vi "ProiectIV.vi"() -> ()   [LabVIEW 2020]
uses:
  65261286-63d7-44c7-95d4-ed37a7534505.vi
  <vilib>/MakerHub/LINX/Public/Peripherals/Digital/Digital Write 1 Chan.vi
  <vilib>/MakerHub/LINX/Public/Peripherals/PWM/PWM Set Duty Cycle 1 Chan.vi
  <vilib>/MakerHub/LINX/Public/Peripherals/Digital/Digital Write N Chans.vi
  <vilib>/MakerHub/LINX/Private/Local IO/LinxDigitalWrite.vi
  <vilib>/MakerHub/LINX/Public/Utilities/Check Channel.vi
  <vilib>/MakerHub/LINX/Public/Utilities/Open Serial.vi
  <vilib>/MakerHub/LINX/Private/Utilties/Generate Error.vi
  <vilib>/MakerHub/LINX/Public/Peripherals/PWM/PWM Set Duty Cycle N Chans.vi
  <vilib>/Comparison/Equal/Equal Functor/Equal Functor.lvclass
  <vilib>/MakerHub/LINX/LMH-LINX.lvlib
panel:
  out "UID Password":string
  out "UID vizibil":string
  out "?":string="Va rugam apropiati cardul"
  out "Nu se permite accesul":bool
  out "Se permite accesul":bool
  in  "Buton de oprire a programului":bool
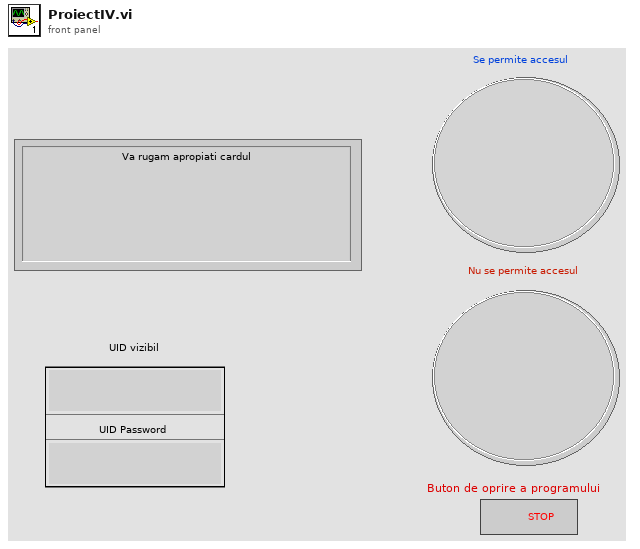
[diagram p1: front panel]
types:
  T1 = typedef "LMH-LINX.lvlib/LINX Ref.ctl" = cluster{"IO":T2, "Interface":T3, "LINX Device Config":T4}
  T2 = typedef "LMH-LINX.lvlib/Platform.ctl" = enum16{"Remote", "Local"}
  T3 = typedef "LMH-LINX.lvlib/Interface.ctl" = enum16{"Serial", "TCP"}
  T4 = typedef "LMH-LINX.lvlib/Device.lvlib/LINX Device Config.ctl" = cluster{"Interface":T3, "COM Port":refnum<visa-resource-name>, "TCP Configuration":T5, "Device Family":u8, "Device ID":u8, "Device Name":string, "TCP Ref":refnum<k5>, "Channels":T6}
  T5 = typedef "LMH-LINX.lvlib/Device.lvlib/TCP Config.ctl" = cluster{"IP Address":string, "Port":u16}
  T6 = typedef "LMH-LINX.lvlib/Channels.ctl" = cluster{"DI":u8[], "DO":u8[], "AI":u8[], "AO":u8[], "PWM":u8[], "QE":u8[], "UART":u8[], "I2C 2":u8[], "SPI":u8[], "CAN":u8[], "Servo":u8[], "AI Ref (V)":dbl, "AI Resolution (Bits)":u8, "AO Ref (V)":dbl, "AO Resolution (Bits)":u8}
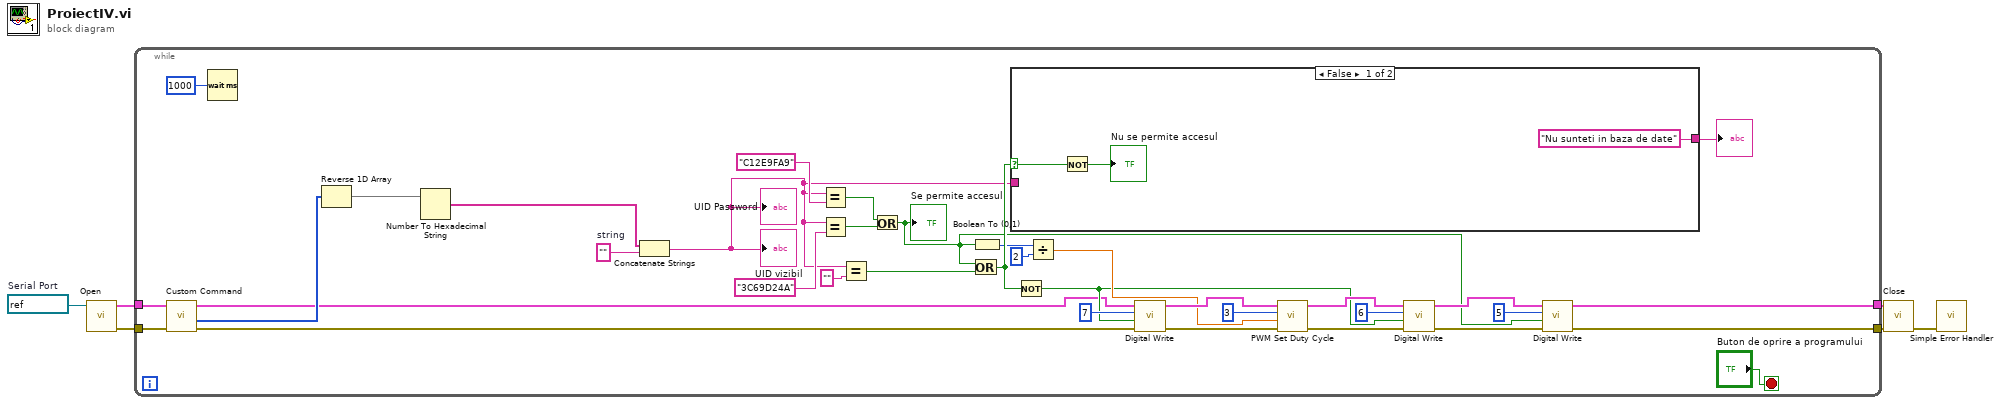
[diagram p0: block diagram]
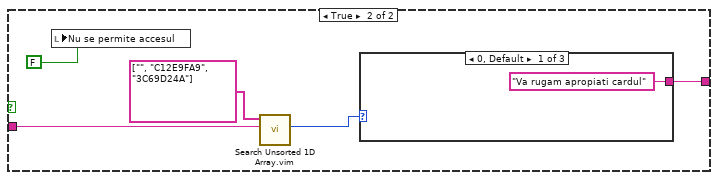
[diagram p2: hidden frame]
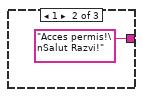
[diagram p3: hidden frame]
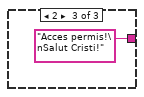
[diagram p4: hidden frame]
diagram:
  w3 = refnum<visa-resource-name> "COM3"  # Serial Port
  n1 = call-poly <vilib>:"Open.vi"("Serial Port"=w3) -> ("Error Out"=w5:errorcluster, "LINX Resource"=w6:T1)  [unwired: 8 in, 1 out]
  n2 = while {
    tunnel: w6 -> [w42]
    tunnel: w5 -> [w41]
    tunnel: [w12] -> w2
    tunnel: [w11] -> w1
    stop <- "Buton de oprire a programului" stop-if-true
    w37 = ""  # string
    n3 = call <vilib>:"Custom Command.vi"("Error In"=w41, "LINX Resource"=w42) -> ("Error Out"=w28:errorcluster, "Response"=w40:u8[], "LINX Resource"=w8:T1)  [unwired: 6 in, 1 out]
    n4 = Wait (ms)(milliseconds to wait=u32 1000) -> ()  [unwired: 1 out]
    n5 = Reverse 1D Array(array=w40) -> (reversed array=w32:u8[])
    n6 = Number To Hexadecimal String(2:w32) -> (0:w38:string[])  [unwired: 1 in]
    n7 = Concatenate Strings "Concatenate Strings"(w38, w37) -> (w7:string)
    "UID vizibil" <- w7
    "UID Password" <- w7
    n8 = Equal?(x=w7, y="C12E9FA9" ("false string")) -> (x = y?=w31:bool)
    n9 = Equal?(x=w7, y="3C69D24A") -> (x = y?=w33:bool)
    n10 = Equal?(x=w7, y="") -> (x = y?=w29:bool)
    n11 = Or(x=w31, y=w33) -> (x .or. y?=w9:bool)
    "Se permite accesul" <- w9
    n12 = Or(x=w9, y=w29) -> (x .or. y?=w26:bool)
    n13 = Boolean To (0,1)(Boolean=w9) -> (0, 1=w21:i16)
    n14 = case shown="False" w26 {
      selector: w26 -> [w43 _]
      tunnel: ["Nu sunteti in baza de date" w48] -> w25
      tunnel: w7 -> [_ w47]
      frame False {
        n15 = Not(x=w43) -> (.not. x?=→"Nu se permite accesul":bool)
      }
      frame True {
        n16 = local write "Nu se permite accesul"(FALSE ("Boolean 3")) -> ()
        n17 = call "Search Unsorted 1D Array.vim"("element"=w47, "unsorted 1D array"=string[] ["", "C12E9FA9", "3C69D24A"]) -> ("index of element"=w49:i32)  [unwired: 9 in]
        n18 = case shown="0, Default" w49 {
          tunnel: ["Va rugam apropiati cardul" "Acces permis!\nSalut Razvi!" "Acces permis!\nSalut Cristi!"] -> w48
          frame 0, Default {
          }
          frame 1 {
          }
          frame 2 {
          }
        }
      }
    }
    "?" <- w25
    n19 = Not(x=w26) -> (.not. x?=w10:bool)
    n20 = Divide(x=w21, y=i16 2) -> (x/y=w19:dbl)
    n21 = call-poly <vilib>:"Digital Write.vi"("Error In"=w28, "Output Value"=w10, "DO Channel"=u8 7, "LINX Resource"=w8) -> ("Error Out"=w22:errorcluster, "LINX Resource"=w23:T1)  [unwired: 6 in]
    n22 = call-poly <vilib>:"PWM Set Duty Cycle.vi"("Error In"=w22, "Duty Cycle (0-1)"=w19, "PWM Channel"=u8 3 ("AO Channel"), "LINX Resource"=w23) -> ("Error Out"=w17:errorcluster, "LINX Resource"=w18:T1)  [unwired: 6 in]
    n23 = call-poly <vilib>:"Digital Write.vi"("Error In"=w17, "Output Value"=w10, "DO Channel"=u8 6, "LINX Resource"=w18) -> ("Error Out"=w15:errorcluster, "LINX Resource"=w16:T1)  [unwired: 6 in]
    n24 = call-poly <vilib>:"Digital Write.vi"("Error In"=w15, "Output Value"=w9, "DO Channel"=u8 5, "LINX Resource"=w16) -> ("Error Out"=w11:errorcluster, "LINX Resource"=w12:T1)  [unwired: 6 in]
  }
  n25 = call <vilib>:"Close.vi"("Error In"=w1, "LINX Resource"=w2) -> ("Error Out"=w4:errorcluster)  [unwired: 9 in]
  n26 = call <vilib>:"Simple Error Handler.vi"("error in (no error)"=w4) -> ()  [unwired: 4 in, 5 out]
